vi "Login.vi"(7 "error in (no error)":errorcluster, 10 "reference in":refnum<class "MES_Local.lvclass">) -> (0 "error out":errorcluster, 1 "Cancelled":bool, 2 "Valid":bool, 3 "reference in":refnum<class "MES_Local.lvclass">)   [LabVIEW 2022 SP3, in "MES_Local.lvlib" / "MES_Local.lvclass"]
uses:
  MES_Local.lvclass
  Components/Login_Base.lvlibp/Login_Base.lvclass
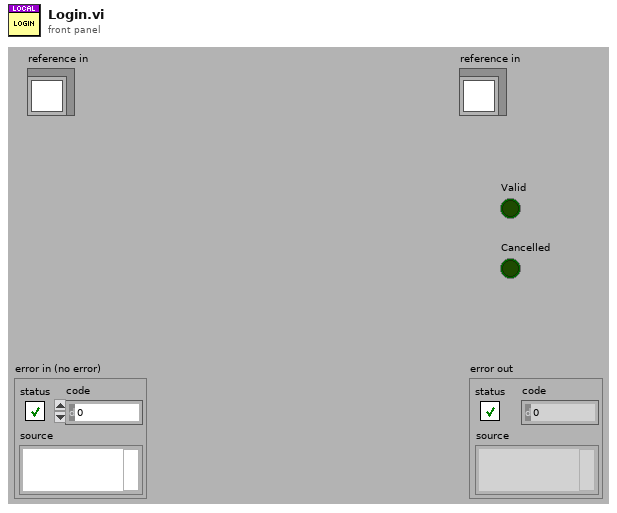
[diagram p1: front panel]
types:
  T1 = typedef "MES_Local.lvlib/MES_Local.lvclass/ObjectAttributes.ctl" = cluster{"Config":T2, "Logged_In?":bool, "AttributeNames":string[], "AttributeWritten":bool[], "ComponentNames":string[], "TestIndex":i32, "TestTag":string[], "Time Stamp":timestamp, "Employee":string, "Resource_Key":string, "Local Spec":path, "Login":refnum<class "Login_Base.lvclass">, "ReportPath":path, "Spec":T3, "StartTime":timestamp, "Role":string}
  T2 = typedef "MES_Local.lvlib/MES_Local.lvclass/Config.ctl" = cluster{"Results_Path":path}
  T3 = typedef "MES_Base.lvlibp/MES_Base.lvclass/Spec.ctl" = cluster{"Header":cluster{"Doctype":string, "Checksum":string, "DriverKey":string, "SpecId":string, "TransactionId":string, "AccountId":string, "SpecName":string, "WorkflowStep":string, "SerialNumber":string, "BatchNumber":string, "Status":enum16{"Pending", "Pass", "Fail"}, "Comment":string, "FirstFail":string, "Employee":string, "LocalMachine":string, "ResourceKey":string, "Date":string, "Time":string, "Duration":string, "DUT Position":i32}, "Components":cluster{"SerialNumber":string, "PartNumber":string, "Revision":string, "BatchNumber":string, "Name":string, "Description":string, "Attached":bool}[], "Attributes":cluster{"Name":string, "Description":string, "DataType":enum16{"NA", "String", "Boolean", "Int", "Dbl"}, "Value":variant, "DisplayFormat":string, "ReadOnly":bool, "Required":bool}[], "Tests":cluster{"Code":string, "Name":string, "Description":string, "Group":string, "IsGroup":bool, "Tag":string, "Method":string, "Parrameter":string, "DataType":enum16{"NA", "String", "Boolean", "Int", "Dbl"}, "Value":variant, "Status":enum16{"Pending", "Pass", "Fail"}, "LimitLo":variant, "LimitHi":variant, "StringMatch":string, "BooleanMatch":bool, "DisplayFormat":string, "Units":string, "TestTime":dbl}[]}
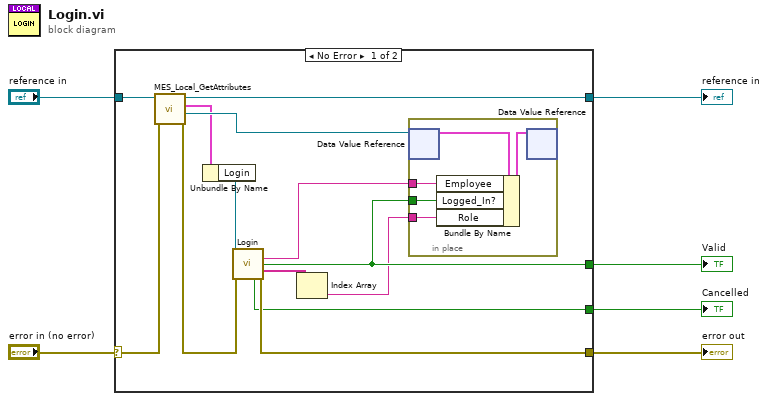
[diagram p0: block diagram]
diagram:
  n1 = case shown="No Error" "error in (no error)" {
    selector: "error in (no error)" -> [w19 w26]
    tunnel: [w12 w26] -> w5
    tunnel: [w17 w25] -> w3
    tunnel: "reference in" -> [w18 w25]
    tunnel: [w9 _] -> w2
    tunnel: [w10 _] -> w1
    frame No Error {
      n2 = call "MES_Local_GetAttributes.vi"("error in (no error)"=w19, "reference in"=w18) -> ("error out"=w13:errorcluster, "DataRef"=w16:refnum<data-value>, "Data"=w15:T1, "reference out"=w17:refnum<class "MES_Local.lvclass">)  [unwired: 6 in]
      n3 = Unbundle By Name(w15) -> ("Login"=w14:refnum<class "Login_Base.lvclass">)
      n4 = call-dynamic "Login.vi"("reference in"=w14, "error in (no error)"=w13) -> ("User"=w11:string, "valid"=w9:bool, "Rights"=w8:string[], "Cancelled"=w10:bool, "error out"=w12:errorcluster)  [unwired: 7 in, 2 out]
      n5 = Index Array(array=w8) -> (element=w7:string)  [unwired: 1 in]
      n6 = in-place {
        in-place-border: w11 -> [w22]
        in-place-border: w9 -> [w21]
        in-place-border: w7 -> [w20]
        n7 = in-place-dvr #1(w16) -> (w24:T1)  [unwired: 1 out]
        n8 = Bundle By Name(cluster=w24, "Employee"=w22, "Logged_In?"=w21, "Role"=w20) -> (w23:T1)
        n9 = in-place-dvr #1(w23) -> ()  [unwired: 2 out]
      }
    }
    frame Error {
    }
  }
  "error out" <- w5
  "reference in" <- w3
  "Valid" <- w2
  "Cancelled" <- w1
